vi "add_system_path.vi"(8 "error in (no error)":errorcluster) -> (0 "error out":errorcluster)   [LabVIEW 2015, in "lv-bin-git.lvlib"]
uses:
  lv-bin-git.lvlib
  private/_controls/file.ctl
  <userlib>/antonio-alexander/lv-bin/public/api/v1/v1.lvlib
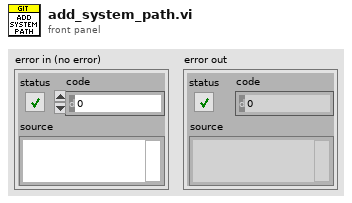
[diagram p1: front panel]
types:
  T1 = typedef "lv-bin-git.lvlib/file.ctl" = enum16{"<file.extension>", "git.exe"}
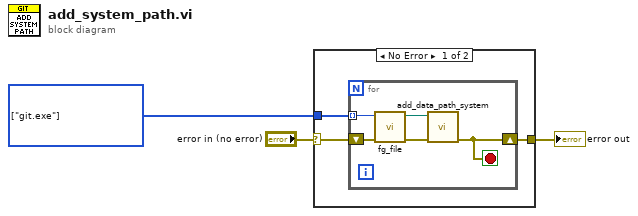
[diagram p0: block diagram]
diagram:
  w3 = T1[] [enum."git.exe"] items=["<file.extension>", "git.exe"]
  n1 = case shown="No Error" "error in (no error)" {
    selector: "error in (no error)" -> [w5 w12]
    tunnel: w3 -> [w6 _]
    tunnel: [w4 w12] -> w1
    frame No Error {
      n2 = for {
        tunnel: w6 -> [w11] mode=indexing
        shift-right: [w8] -> w4
        shift-left: w5 -> [w10]
        stop <- w8 stop-if-true
        n3 = call "fg_file.vi"("error in (no error)"=w10, "file"=w11) -> ("error out"=w9:errorcluster, "filename"=w7:path)  [unwired: 8 in]
        n4 = call <userlib>:"add_data_path_system.vi"("error in (no error)"=w9, "relative_path_file"=w7) -> ("error out"=w8:errorcluster)  [unwired: 9 in]
      }
    }
    frame Error {
    }
  }
  "error out" <- w1
